vi "Go To Do Nothing Command.vi"(8 "error in (no error)":errorcluster, 11 "Receiver Commands in":refnum<class "Receiver Command.lvclass">) -> (0 "error out":errorcluster, 3 "State out":refnum<class "State Actor.lvclass">)   [LabVIEW 2013, in "Receiver.lvlib" / "Receive Commands Using State Actors.lvlib" / "Receiver Command.lvclass"]
uses:
  Receiver Command.lvclass
  <vilib>/ni/Actors/State Actor/State Actor/State Actor.lvclass
  Do Nothing Command/Do Nothing.lvclass
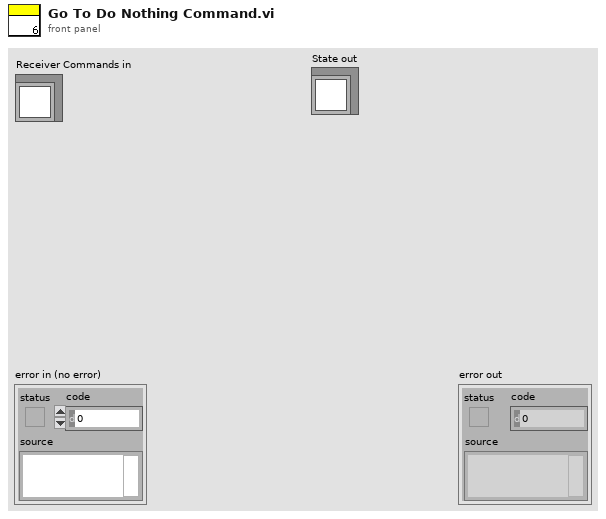
[diagram p1: front panel]
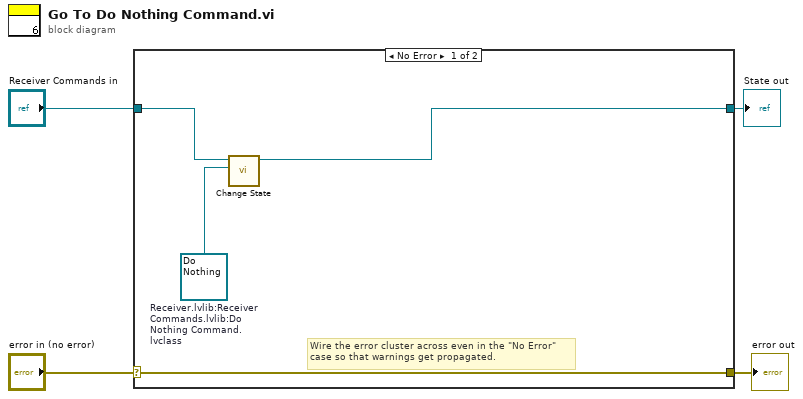
[diagram p0: block diagram]
diagram:
  n1 = case shown="No Error" "error in (no error)" {
    selector: "error in (no error)" -> [w8 w10]
    tunnel: [w8 w10] -> w3
    tunnel: [w5 w9] -> w1
    tunnel: "Receiver Commands in" -> [w6 w9]
    frame No Error {
      w7 = refnum<class "Do Nothing.lvclass"> refnum  # Receiver.lvlib:Receiver Commands.lvlib:Do Nothing Command.lvclass
      # "Wire the error cluster across even in the \"No Error\"\ncase so that warnings get propagated."
      n2 = call <vilib>:"Change State.vi"("New State in"=w7, "State in"=w6) -> ("State out"=w5:refnum<class "State Actor.lvclass">)  [unwired: 8 in, 1 out]
    }
    frame Error {
    }
  }
  "error out" <- w3
  "State out" <- w1
